vi "Ohaus AV Series Interactive Measurement.vi"() -> ()   [LabVIEW 2015]
doc: "This VI initializes the balance with default settings, then takes a measurement every time the \"Take Measurement\" button is pressed. The value is then added to the Array and the Chart so that a record of the data can be kept.\n\n<B>Before running this VI some initial instrument setup is required:</B>\nOnly Gross, Net, Tare; Reference; and GLP need to be changed from their default values to OFF\n\nGoto the menu screen on the balance\n Then the PRINT-1 menu\n \n Output\n When Stable: OFF (default) \n GLP Tare: OFF (default)\n Auto Print: OFF (default)\n Content\n Number Only: OFF (default)\n Header: OFF (default)\n<B> Gross, Net, and Tare: OFF</B>\n<B> Reference: OFF</B>\n Result: ON (default)\n<B> GLP: OFF</B>\n Layout\n Line Format: MULTI (default)\n Line Feed: OFF (default)\n Form Feed: OFF (default)"
uses:
  <instrlib>/Ohaus AV Series/Ohaus AV Series.lvlib
panel:
  in  "Serial Configuration":T1={"Baud Rate (2400)"=2400, "Flow Control (1: XON/XOFF)"=1, "Parity (0: None)"=0, "Data Bits (7)"=7} {"Data Bits (7)" items=["7"=7, "8"=8]; "Parity (0: None)" items=["None", "Odd", "Even"]; "Flow Control (1: XON/XOFF)" items=["None", "XON/XOFF", "RTS/CTS"]; "Baud Rate (2400)" items=["600"=600, "1200"=1200, "2400"=2400, "4800"=4800, "9600"=9600, "19200"=19200]}
  in  "VISA resource name":refnum<visa-resource-name>
  in  "Units (0: Gram)":u16(ring) items=["Gram (g)"=0, "Kilogram (kg)"=1, "Penny weight (dwt)"=2, "Carat (ct)"=3, "Ounce (oz)"=4, "Ounce Troy (oz t)"=5, "Grain (GN)"=6, "Hong Kong Tael (HKt)"=7, "Singapore Tael (SGt)"=8, "Tiwan Tael (TWt)"=9, "Momme (m)"=10, "Pound (lb)"=11, "Newton (N)"=13, "Tical (ti)"=14, "Tula"=15, "Mesghal (Meshg)"=16, "Baht"=17, "Custom"=19]
  out "Value Chart":dbl(graph)
  in  "stop":bool
  out "Value Array":dbl[](array[numeric])
  in  "Take Measurement":bool
  # "(c) 2004-2009 National Instruments.  All Rights Reserved."
  # "Before running this VI some initial setup is required\n(See VI documentation for more information)"
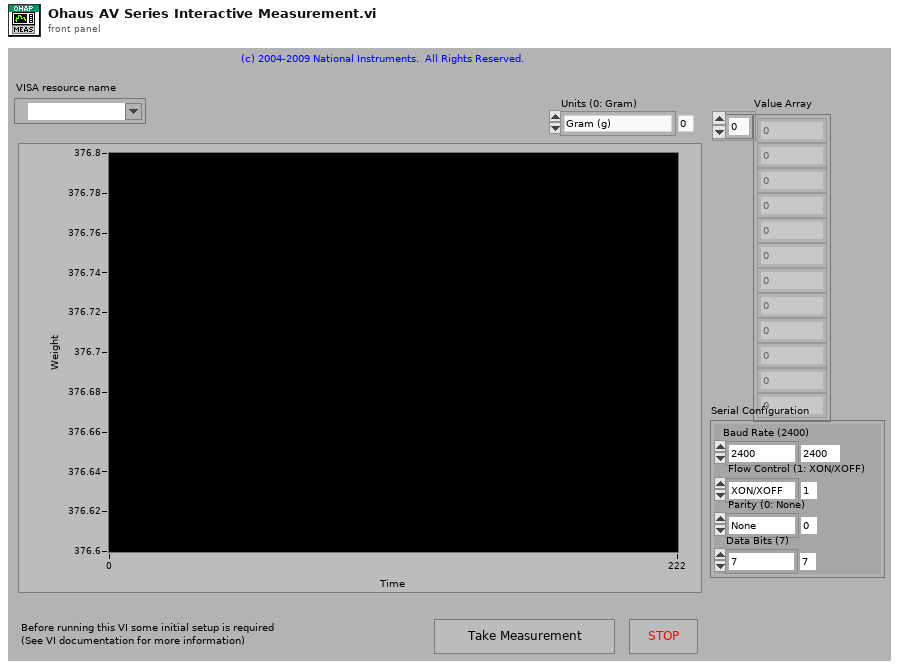
[diagram p1: front panel]
types:
  T1 = cluster{"Baud Rate (2400)":u32, "Flow Control (1: XON/XOFF)":u16, "Parity (0: None)":u16, "Data Bits (7)":u16}
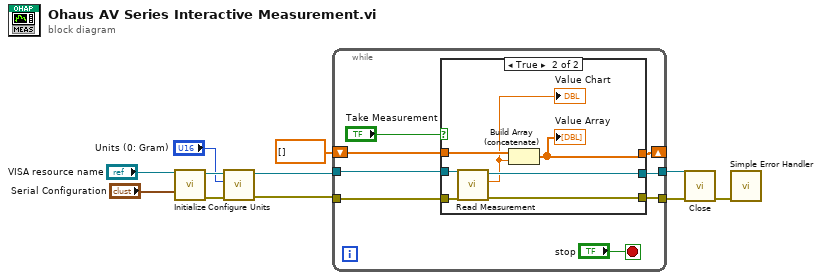
[diagram p0: block diagram]
diagram:
  n1 = call <instrlib>:"Initialize.vi"("VISA resource name"="VISA resource name", "Serial Configuration"="Serial Configuration") -> ("VISA resource name out"=w4:refnum<visa-resource-name>, "error out"=w7:errorcluster)  [unwired: 12 in]
  n2 = call <instrlib>:"Configure Units.vi"("error in (no error)"=w7, "Units (0: Gram)"="Units (0: Gram)", "VISA resource name"=w4) -> ("error out"=w6:errorcluster, "VISA resource name out"=w5:refnum<visa-resource-name>)  [unwired: 7 in]
  n3 = while {
    shift-right: [w16] -> _
    shift-left: dbl[] [] -> [w17]
    tunnel: w5 -> [w19]
    tunnel: [w13] -> w10
    tunnel: w6 -> [w18]
    tunnel: [w12] -> w9
    stop <- "stop" stop-if-true
    n4 = case shown="True" "Take Measurement" {
      tunnel: w19 -> [w21 w29]
      tunnel: w18 -> [w20 w28]
      tunnel: w17 -> [w22 w24]
      tunnel: [w22 w25] -> w16
      tunnel: [w21 w27] -> w13
      tunnel: [w20 w26] -> w12
      frame False {
      }
      frame True {
        n5 = call <instrlib>:"Read Measurement.vi"("error in (no error)"=w28, "VISA resource name"=w29) -> ("error out"=w26:errorcluster, "Weight Value"=w23:dbl, "VISA resource name out"=w27:refnum<visa-resource-name>)  [unwired: 4 in, 3 out]
        "Value Chart" <- w23
        n6 = Build Array (concatenate)(w24, w23) -> (w25:dbl[])
        "Value Array" <- w25
      }
    }
  }
  n7 = call <instrlib>:"Close.vi"("error in (no error)"=w9, "VISA resource name"=w10) -> ("error out"=w8:errorcluster)  [unwired: 9 in]
  n8 = call <vilib>:"Simple Error Handler.vi"("error in (no error)"=w8) -> ()  [unwired: 4 in, 5 out]
